vi "Core.vi"(10 "CMD":refnum<queue>, 11 "Instr in":refnum<class "CRDS.lvclass">=refnum) -> ()   [LabVIEW 2014, in "CRDS.lvclass"]
uses:
  CRDS.lvclass
  Instrument/state.ctl
  Instrument/Instrument.lvclass
  Command/Command.lvclass
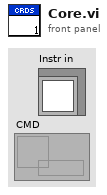
[diagram p1: front panel]
types:
  T1 = typedef "Instrument.lvclass/state.ctl" = enum8{"Configure", "Acquire", "Wait", "Quit", "Handle Error", "NOOP"}
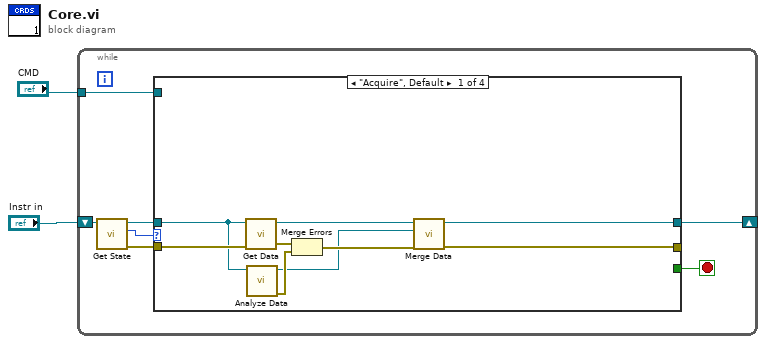
[diagram p0: block diagram]
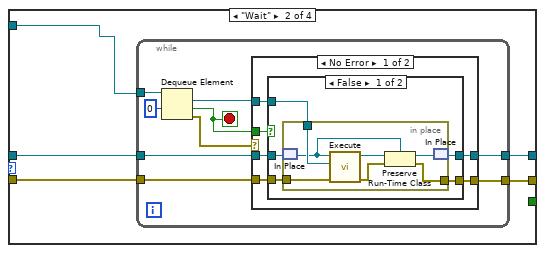
[diagram p2: hidden frame]
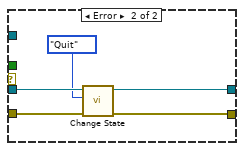
[diagram p4: hidden frame]
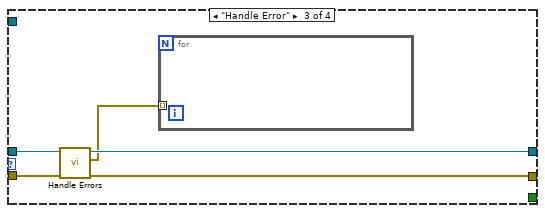
[diagram p5: hidden frame]
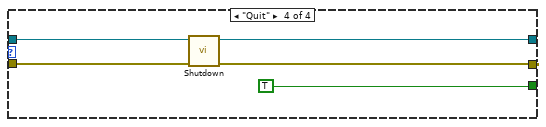
[diagram p6: hidden frame]
diagram:
  n1 = while "Acquisition" {
    shift-right: [w4] -> _
    shift-left: "Instr in" -> [w8]
    tunnel: "CMD" -> [w3]
    stop <- w5 stop-if-true
    n2 = call "Get State.vi"("Instrument in"=w8) -> ("error out"=w6:errorcluster, "default state"=w9:T1, "Instrument out"=w7:refnum<class "Instrument.lvclass">)  [unwired: 8 in]
    n3 = case shown="\"Acquire\", Default" w9 {
      tunnel: w7 -> [w17 w23 w62 w66]
      tunnel: w6 -> [w18 w20 w61 w65]
      tunnel: [_ _ _ TRUE] -> w5
      tunnel: [w13 w22 w59 w64] -> w4
      tunnel: [w11 w21 w60 w63] -> _
      tunnel: w3 -> [_ w19 _ _]
      frame "Acquire", Default {
        n4 = call-dynamic "Get Data.vi"("error in"=w18, "Instrument in"=w17) -> ("error out"=w16:errorcluster, "Instrument out"=w14:refnum<class "Instrument.lvclass">)  [unwired: 8 in]
        n5 = call-dynamic "Analyze Data.vi"("Instrument in"=w17) -> ("error out"=w15:errorcluster, "Instrument out"=w10:refnum<class "Instrument.lvclass">)  [unwired: 9 in]
        n6 = Merge Errors(w16, w15) -> (w12:errorcluster)
        n7 = call-dynamic "Merge Data.vi"("error in"=w12, "Analyzed"=w10, "Acquired"=w14) -> ("error out"=w11:errorcluster, "Instrument out"=w13:refnum<class "Instrument.lvclass">)  [unwired: 7 in]
      }
      frame "Wait" {
        n8 = while {
          tunnel: w19 -> [w32]
          tunnel: w23 -> [w31]
          tunnel: [w30] -> w22
          tunnel: [w28] -> w21
          tunnel: w20 -> [w27]
          stop <- w26 stop-if-true
          n9 = Dequeue Element(queue=w32, timeout in ms (-1)=0) -> (element=w29:refnum<class "Command.lvclass">, timed out?=w26:bool, error out=w25:errorcluster)  [unwired: 1 in, 1 out]
          n10 = case shown="No Error" w25 {
            tunnel: w31 -> [w38 w57]
            tunnel: [w37 w56] -> w30
            tunnel: w29 -> [w36 _]
            tunnel: [w35 w55] -> w28
            tunnel: w27 -> [w34 w54]
            tunnel: w26 -> [w33 _]
            frame No Error {
              n11 = case shown="False" w33 {
                tunnel: w38 -> [w43 w51]
                tunnel: [w42 w51] -> w37
                tunnel: w36 -> [w41 _]
                tunnel: [w40 w52] -> w35
                tunnel: w34 -> [w39 w52]
                frame False {
                  n12 = in-place {
                    in-place-border: w41 -> [w50]
                    in-place-border: [w45] -> w40
                    in-place-border: w39 -> [w44]
                    n13 = in-place-match #1(w43) -> (w49:refnum<class "Instrument.lvclass">)
                    n14 = call "Execute.vi"("error in"=w44, "Command in"=w50, "Object In"=w49) -> ("error out"=w46:errorcluster, "Object Out"=w48:refnum<class>)  [unwired: 7 in]
                    n15 = Preserve Run-Time Class(object in=w48, error in=w46, 2:w49) -> (object out=w47:refnum<class "Instrument.lvclass">, error out=w45:errorcluster)
                    n16 = in-place-match #1(w47) -> (w42:refnum<class "Instrument.lvclass">)
                  }
                }
                frame True {
                }
              }
            }
            frame Error {
              n17 = call "Change State.vi"("error in"=w54, "instr state"=state."Quit", "Instrument in"=w57) -> ("error out"=w55:errorcluster, "Instrument out"=w56:refnum<class "Instrument.lvclass">)  [unwired: 7 in]
            }
          }
        }
      }
      frame "Handle Error" {
        n18 = call-dynamic "Handle Errors.vi"("error in"=w61, "Instrument in"=w62) -> ("error out"=w60:errorcluster, "errors"=w58:errorcluster[], "Instrument out"=w59:refnum<class "Instrument.lvclass">)  [unwired: 7 in]
        n19 = for {
          tunnel: w58 -> [_] mode=indexing
        }
      }
      frame "Quit" {
        n20 = call-dynamic "Shutdown.vi"("error in"=w65, "Instrument in"=w66) -> ("error out"=w63:errorcluster, "Instrument out"=w64:refnum<class "Instrument.lvclass">)  [unwired: 8 in]
      }
    }
  }
